vi "Create Log File.vi"(8 "error in (no error)":errorcluster, 11 "appended path":path) -> (0 "error out":errorcluster, 3 "Refnum out":refnum<k34>)   [LabVIEW 2020, in "Mock LC Parser.lvlib" / "Logging.lvlib"]
uses:
  Logging.lvlib
panel:
  in  "Log File Type":string="CSV"
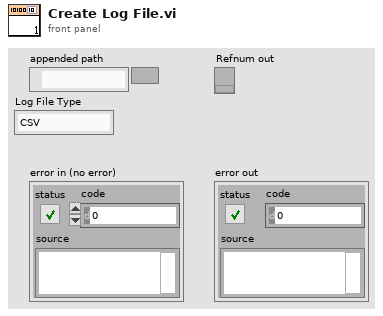
[diagram p1: front panel]
types:
  T1 = enum16{"open", "replace", "create", "open or create", "replace or create", "replace or create with confirmation"}
  T2 = enum16{"open", "open or create", "create or replace", "create", "open (read-only)"}
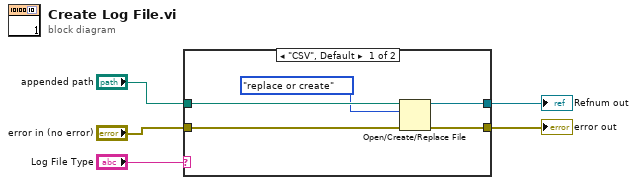
[diagram p0: block diagram]
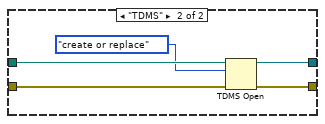
[diagram p2: hidden frame]
diagram:
  n1 = case shown="\"CSV\", Default" "Log File Type" {
    tunnel: "error in (no error)" -> [w9 w15]
    tunnel: [w7 w14] -> w4
    tunnel: [w6 w13] -> w3
    tunnel: "appended path" -> [w10 w12]
    frame "CSV", Default {
      n2 = Open/Create/Replace File(file path (use dialog)=w10, error in=w9, operation (0:open)=T1."replace or create") -> (refnum out=w7:refnum<file>, error out=w6:errorcluster)  [unwired: 3 in, 1 out]
    }
    frame "TDMS" {
      n3 = TDMS Open(8:w15, 10:T2."create or replace" ("operation (0:open)"), 11:w12) -> (0:w13:errorcluster, 3:w14:refnum<k34>)  [unwired: 4 in]
    }
  }
  "Refnum out" <- w4
  "error out" <- w3
